vi "Test (Replace 2D Array in Default JSON).vi"(8 "error in (no error)":errorcluster, 11 "VCluster with Array of Arrays":variant=variant(cluster{"InitialCluster":cluster{"Array":variant[]}} {"InitialCluster"={"Array"=[variant(cluster{"Name":string, "Dept":string, "2DArray":variant[]} {"Name"="S.Raakesh", "Dept"="E", "2DArray"=[variant(variant[] [variant(u64 1), variant(u64 2)]), variant(variant[] [variant(u64 3), variant(u64 4)])]}), variant(cluster{"Name":string, "Dept":string, "2DArray":variant[]} {"Name"="1ABC2", "Dept"="E", "2DArray"=[variant(variant[] [variant(u64 1), variant(u64 2)]), variant(variant[] [variant(u64 3), variant(u64 4)])]})]}})) -> (0 "error out":errorcluster, 3 "VCluster with replaced 2D Array":variant)   [LabVIEW 2015]
uses:
  <vilib>/Utility/Data Type/NI_Data Type.lvlib
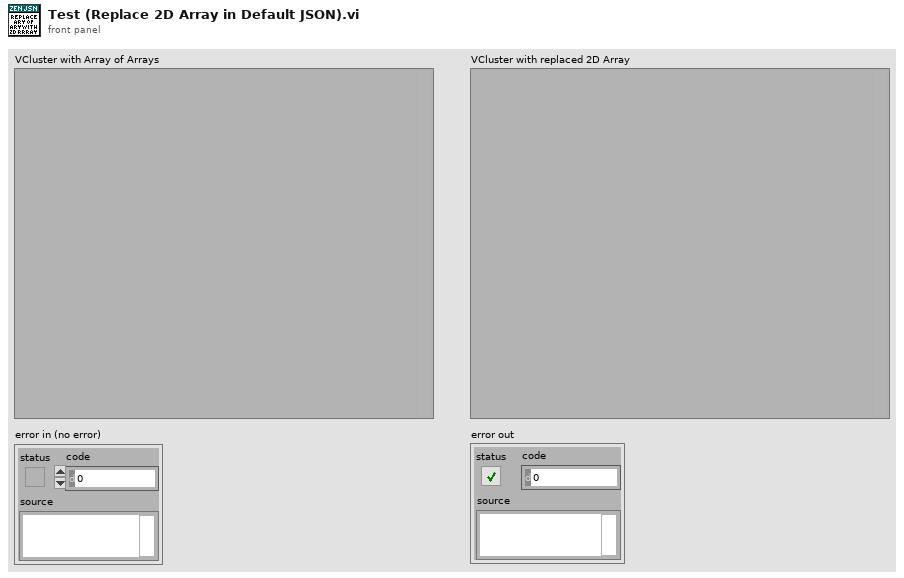
[diagram p1: front panel]
types:
  T1 = typedef "NI_Data Type.lvlib/Data Type.ctl" = enum8{"Invalid Type", "Void", "I8", "I16", "I32", "I64", "U8", "U16", "U32", "U64", "Single Float", "Double Float", "Extended Float", "Single Complex", "Double Complex", "Extended Complex", "Enum U8", "Enum U16", "Enum U32", "Enum U64", "Single Float With Unit", "Double Float With Unit", "Extended Float With Unit", "Single Complex with Unit", "Double Complex with Unit", "Extended Complex with Unit", "Boolean", "String", "Path", "Picture", "Tag", "Array", "Cluster", "Variant", "LV Variant", "Waveform", "Timestamp", "Digital Waveform", "Digital Data", "ExpressData", "Refnum", "External Data", "VI", "Poly VI", "LabVIEW Class Instance", "Fixed Point"}
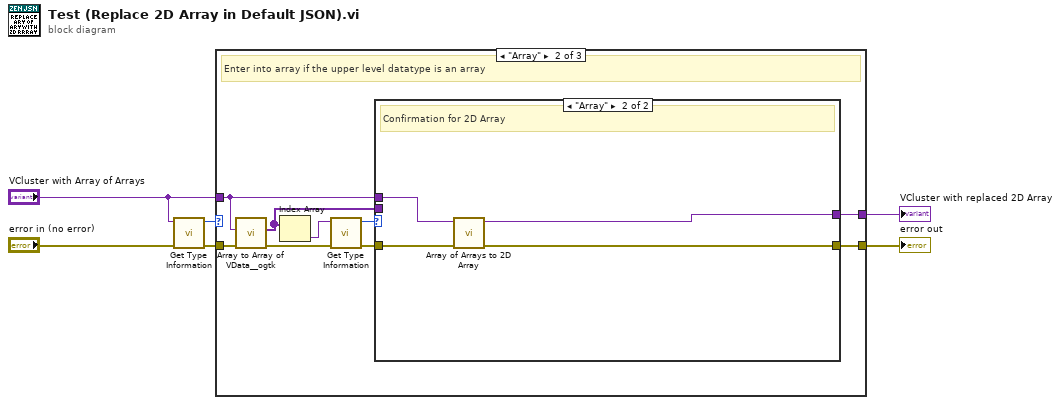
[diagram p0: block diagram]
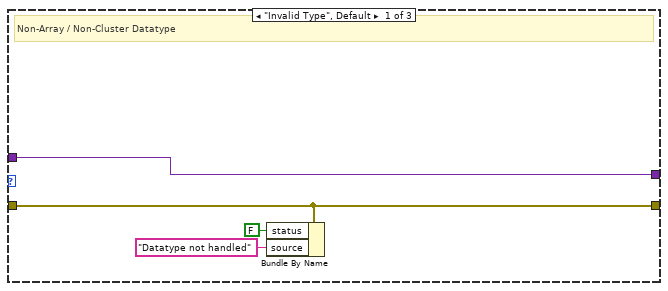
[diagram p2: hidden frame]
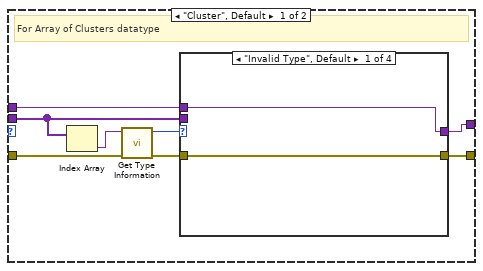
[diagram p3: hidden frame]
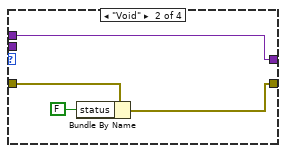
[diagram p4: hidden frame]
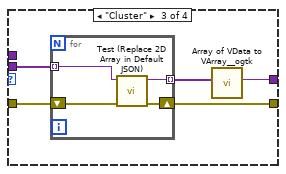
[diagram p5: hidden frame]
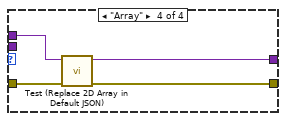
[diagram p6: hidden frame]
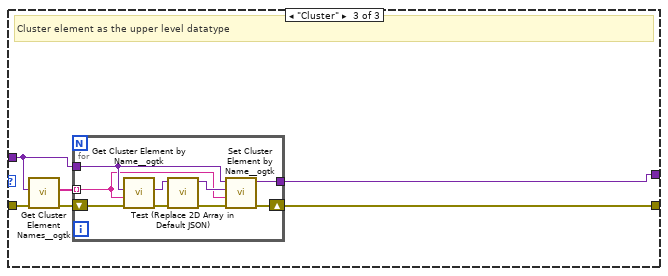
[diagram p7: hidden frame]
diagram:
  n1 = call <vilib>:"Get Type Information.vi"("error in (no error)"="error in (no error)", "Variant"="VCluster with Array of Arrays") -> ("error out"=w5:errorcluster, "Type"=w6:T1)  [unwired: 5 in, 3 out]
  n2 = case shown="\"Array\"" w6 {
    tunnel: "VCluster with Array of Arrays" -> [w10 w17 w55]
    tunnel: w5 -> [w7 w15 w54]
    tunnel: [w10 w18 w52] -> w3
    tunnel: [w7 w19 w51] -> w2
    frame "Invalid Type", Default {
      # "Non-Array / Non-Cluster Datatype"
      n3 = Bundle By Name(cluster=w7, "status"=FALSE, "source"="Datatype not handled") -> ()  [unwired: 1 out]
    }
    frame "Array" {
      # "Enter into array if the upper level datatype is an array"
      n4 = call <userlib>:"Array to Array of VData__ogtk.vi"("error in (no error)"=w15, "MultiD Array"=w17) -> ("error out"=w14:errorcluster, "1D Array of Variants"=w11:variant[])  [unwired: 8 in]
      n5 = Index Array(array=w11) -> (element=w12:variant)  [unwired: 1 in]
      n6 = call <vilib>:"Get Type Information.vi"("error in (no error)"=w14, "Variant"=w12) -> ("error out"=w13:errorcluster, "Type"=w16:T1)  [unwired: 5 in, 3 out]
      n7 = case shown="\"Array\"" w16 {
        tunnel: w13 -> [w23 w49]
        tunnel: [w26 w47] -> w19
        tunnel: [w25 w50] -> w18
        tunnel: w17 -> [w22 w48]
        tunnel: w11 -> [w20 _]
        frame "Cluster", Default {
          # "For Array of Clusters datatype"
          n8 = Index Array(array=w20) -> (element=w24:variant)  [unwired: 1 in]
          n9 = call <vilib>:"Get Type Information.vi"("error in (no error)"=w23, "Variant"=w24) -> ("error out"=w21:errorcluster, "Type"=w27:T1)  [unwired: 5 in, 3 out]
          n10 = case shown="\"Invalid Type\", Default" w27 {
            tunnel: w20 -> [_ _ w38 _]
            tunnel: [w29 w33 w36 w45] -> w25
            tunnel: w22 -> [w29 w33 _ w46]
            tunnel: w21 -> [w28 w32 w34 w44]
            tunnel: [w28 w30 w35 w43] -> w26
            frame "Invalid Type", Default {
            }
            frame "Void" {
              n11 = Bundle By Name(cluster=w32, "status"=FALSE) -> (w30:errorcluster)
            }
            frame "Cluster" {
              n12 = for {
                tunnel: w38 -> [w42] mode=indexing
                tunnel: [w41] -> w37 mode=indexing
                shift-right: [w40] -> w35
                shift-left: w34 -> [w39]
                n13 = call "Test (Replace 2D Array in Default JSON).vi"("error in (no error)"=w39, "VCluster with Array of Arrays"=w42) -> ("error out"=w40:errorcluster, "VCluster with replaced 2D Array"=w41:variant)  [unwired: 8 in]
              }
              n14 = call <userlib>:"Array of VData to VArray__ogtk.vi"("1D Array of VData"=w37) -> ("VArray"=w36:variant)  [unwired: 9 in, 1 out]
            }
            frame "Array" {
              n15 = call "Test (Replace 2D Array in Default JSON).vi"("error in (no error)"=w44, "VCluster with Array of Arrays"=w46) -> ("error out"=w43:errorcluster, "VCluster with replaced 2D Array"=w45:variant)  [unwired: 8 in]
            }
          }
        }
        frame "Array" {
          # "Confirmation for 2D Array"
          n16 = call "Array of Arrays to 2D Array.vi"("error in (no error)"=w49, "Variant in"=w48) -> ("error out"=w47:errorcluster, "Variant out"=w50:variant)  [unwired: 7 in, 1 out]
        }
      }
    }
    frame "Cluster" {
      # "Cluster element as the upper level datatype"
      n17 = call <userlib>:"Get Cluster Element Names__ogtk.vi"("error in (no error)"=w54, "Cluster"=w55) -> ("error out"=w53:errorcluster, "Element Names"=w56:string[])  [unwired: 8 in]
      n18 = for {
        tunnel: w56 -> [w58] mode=indexing
        tunnel: w55 -> [w59]
        shift-right: [w61] -> w51
        shift-left: w53 -> [w65]
        tunnel: [w57] -> w52
        n19 = call <userlib>:"Get Cluster Element by Name__ogtk.vi"("error in (no error)"=w65, "Element Name"=w58, "Cluster"=w59) -> ("error out"=w64:errorcluster, "VElement"=w63:variant)  [unwired: 6 in, 1 out]
        n20 = call "Test (Replace 2D Array in Default JSON).vi"("error in (no error)"=w64, "VCluster with Array of Arrays"=w63) -> ("error out"=w62:errorcluster, "VCluster with replaced 2D Array"=w60:variant)  [unwired: 8 in]
        n21 = call <userlib>:"Set Cluster Element by Name__ogtk.vi"("error in (no error)"=w62, "Element Name (\"\": New Element Data Name)"=w58, "New Element Value"=w60, "Cluster"=w59) -> ("error out"=w61:errorcluster, "VCluster out"=w57:variant)  [unwired: 5 in, 1 out]
      }
    }
  }
  "VCluster with replaced 2D Array" <- w3
  "error out" <- w2
